vi "testcase - Get INI-Static-Variable with Cache.vi"() -> ()   [LabVIEW 2017]
uses:
  INI-Static-Variable-Support/INI-Static-Variable-Support.lvlib
  INI-Static-Variable-Support/_Support/global-csm-ini-db-change-flag.vi
panel:
  in  "String out 2":string="www.openlab.com"
  in  "Boolean":bool
  out "csm-ini-db-change-flag":u32
  in  "stop":bool
  out "Key Found?":bool
  out "String out":string
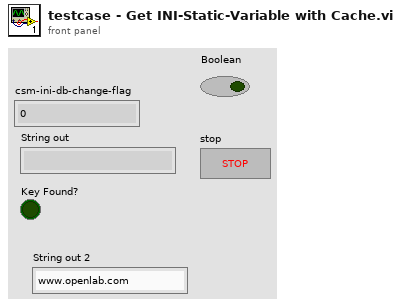
[diagram p1: front panel]
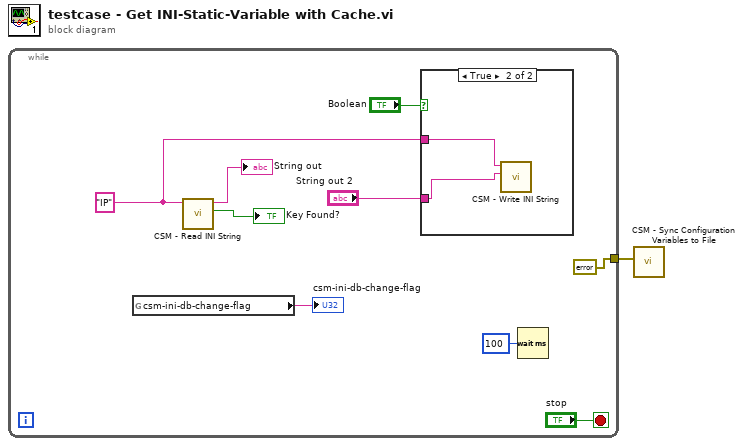
[diagram p0: block diagram]
diagram:
  n1 = while {
    tunnel: [errorcluster {"status"=FALSE, "code"=0, "source"=""} ("error in (no error)")] -> w1
    stop <- "stop" stop-if-true
    w3 = "IP" ("String in")
    n2 = global read "global-csm-ini-db-change-flag.vi" "csm-ini-db-change-flag"() -> (→"csm-ini-db-change-flag":string)
    n3 = call "CSM - Read INI String.vi"("String in"=w3) -> ("Key Found?"=→"Key Found?":bool, "String out"=→"String out":string)  [unwired: 6 in, 1 out]
    n4 = case shown="True" "Boolean" {
      tunnel: w3 -> [_ w12]
      tunnel: "String out 2" -> [_ w11]
      frame False {
      }
      frame True {
        n5 = call "CSM - Write INI String.vi"("String"=w11, ">> Variable Name >>"=w12) -> ()  [unwired: 6 in, 2 out]
      }
    }
    n6 = Wait (ms)(milliseconds to wait=u32 100) -> ()  [unwired: 1 out]
  }
  n7 = call "CSM - Sync Configuration Variables to File.vi"("error in (no error)"=w1) -> ()  [unwired: 8 in, 1 out]
